vi "Motor Stop.vi"(8 "error in (no error)":errorcluster, 11 "Grove I2C L298P Motor Drive in":refnum<class "Grove I2C L298P Motor Drive.lvclass">) -> (0 "error out":errorcluster, 3 "Grove I2C L298P Motor Drive out":refnum<class "Grove I2C L298P Motor Drive.lvclass">)   [LabVIEW 2020, in "CTI-Peripheral.lvlib" / "Grove I2C L298P Motor Drive.lvclass"]
uses:
  Grove I2C L298P Motor Drive.lvclass
  Grove I2C L298P Motor Drive.lvclass/Grove I2C L298P Motor Drive.ctl
  CTI/I2C Connection/I2C Connection.lvclass/I2C Connection.ctl
  CTI/Session/I2C Write Data.vi
  CTI/I2C Connection/I2C Connection.lvclass
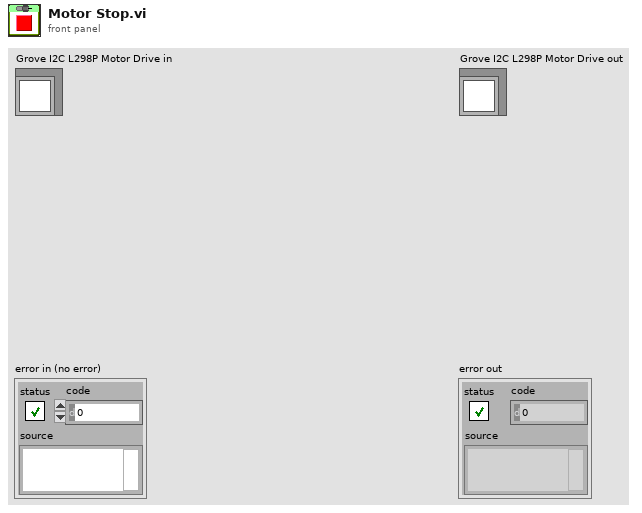
[diagram p1: front panel]
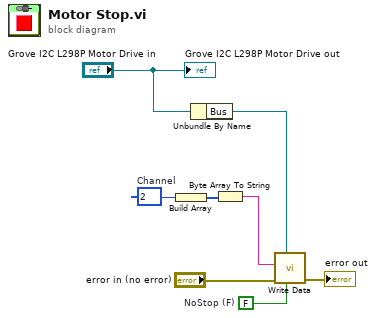
[diagram p0: block diagram]
diagram:
  w4 = u8 2  # Channel
  w5 = FALSE  # NoStop (F)
  n1 = Build Array(w4) -> (w3:u8[])
  n2 = Unbundle By Name("Grove I2C L298P Motor Drive in") -> ("Bus"=w6:refnum<class "I2C Connection.lvclass">)
  n3 = Byte Array To String(unsigned byte array=w3) -> (string=w1:string)
  n4 = call "Write Data.vi"("NoStop (F)"=w5, "I2C Connection"=w6, "error in (no error)"="error in (no error)", "Data"=w1) -> ("error out"=→"error out":errorcluster)  [unwired: 7 in]
  "Grove I2C L298P Motor Drive out" <- "Grove I2C L298P Motor Drive in"
